vi "get_firmware_version.vi"(8 "error in (no error)":errorcluster, 11 "Modbus Master in":refnum<class "Modbus Master.lvclass">) -> (0 "error out":errorcluster, 2 "Firmware version":string, 3 "Modbus Master out":refnum<class "Modbus Master.lvclass">)   [LabVIEW 2018, in "ICP xET-7017.lvlib"]
uses:
  ICP xET-7017.lvlib
  <vilib>/NI/Modbus Library/API/Master/Modbus Master.lvclass
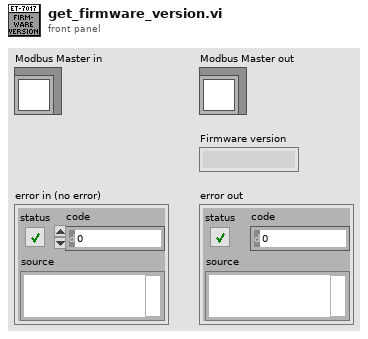
[diagram p1: front panel]
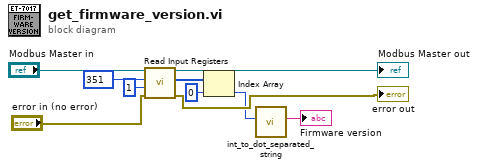
[diagram p0: block diagram]
diagram:
  n1 = call-dynamic "Read Input Registers.vi"("error in"="error in (no error)", "number of inputs"=u16 1, "starting address"=u16 351, "Modbus master in"="Modbus Master in") -> ("error out"=→"error out":errorcluster, "register values"=w3:u16[], "Modbus master out"=→"Modbus Master out":refnum<class "Modbus Master.lvclass">)  [unwired: 5 in]
  n2 = Index Array(array=w3, index=0) -> (element=w5:u16)
  n3 = call "int_to_dot_separated_string.vi"("integer"=w5) -> ("dot fmt string"=→"Firmware version":string)  [unwired: 10 in]
